vi "Load Settings from XML.vi"(8 "error in (no error)":errorcluster, 11 "Settings in":T1 {"Processing Settings"."Test Parameters"."Allowed Tolerance (%) FS" format="%#_4g"; "Acq Settings"."Config Settings"."Simulated Sensor Injection" scale=0.0..100.0}) -> (0 "error out":errorcluster, 3 "Settings out":T1 {"Processing Settings"."Test Parameters"."Allowed Tolerance (%) FS" format="%#_4g"; "Acq Settings"."Config Settings"."Simulated Sensor Injection" scale=0.0..100.0})   [LabVIEW 2026, in "Settings.lvlib"]
doc: "Attempts to load previous user specified settings from an XML file.\n\nThis VI will not generate an error. If a suitable XML file can't be loaded and parsed then it will simply return the default settings."
uses:
  Settings.lvlib
  <vilib>/Utility/xml.llb/Read From XML File(string).vi
  <vilib>/Utility/xml.llb/Write to XML File(string).vi
  Acquisition/Instrument Specifications Configuration.ctl
  Acquisition/Acquisition.lvlib
  controls/UI/Settings Cluster.ctl
  controls/UI/Measurement Role.ctl
  Acquisition/Instrument Specifications Cluster Configuration.ctl
  controls/UI/Config Settings.ctl
  controls/UI/Acq Settings.ctl
  controls/UI/Units Enum.ctl
  controls/UI/Signal Enum.ctl
  controls/Messaging Payloads/Sensor CoreData Cluster.ctl
  controls/Messaging Payloads/Sensor CoreData.ctl
  Processing/Test Parameters Cluster.ctl
  Processing/Test Parameters.ctl
  Processing/Processing_Engine.lvlib
  controls/UI/Direction.ctl
  controls/UI/Test Sequence Context Cluster.ctl
  controls/UI/Test Sequence Context.ctl
  Processing/Processing Settings.ctl
  controls/UI/Session Identfiers.ctl
  controls/UI/Test Sequence Enum.ctl
  controls/UI/Test Sequence State.ctl
  controls/UI/Test Sequence Settings.ctl
  controls/Controller/Controller Core Data.ctl
  controls/Controller/Stimulus Role.ctl
  controls/Controller/Stimulus Output Configuration.ctl
  controls/Controller/Stimulus Output.ctl
  controls/Controller/Stimulus Outputs.ctl
  controls/Controller/Stimulus Settings.ctl
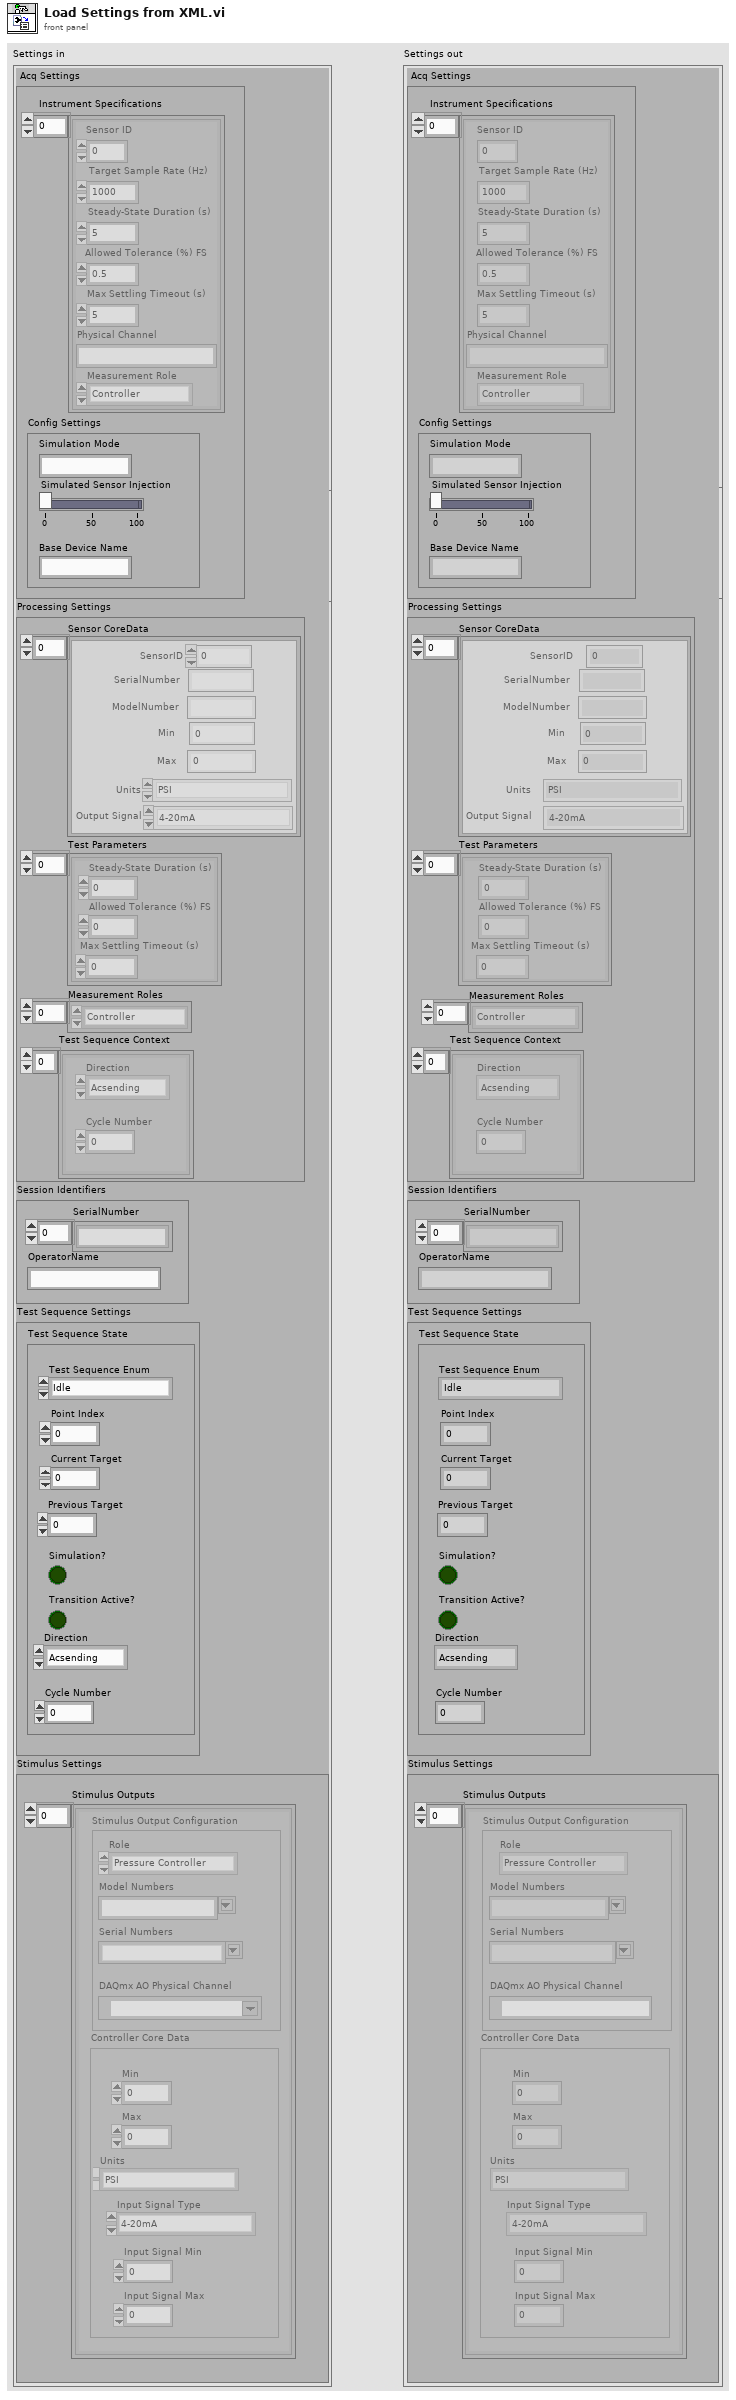
[diagram p1: front panel]
types:
  T1 = typedef "Settings Cluster.ctl" = cluster{"Acq Settings":T2, "Processing Settings":T7, "Session Identifiers":T17, "Test Sequence Settings":T18, "Stimulus Settings":T21}
  T2 = typedef "Acq Settings.ctl" = cluster{"Instrument Specifications":T3, "Config Settings":T6}
  T3 = typedef "Acquisition.lvlib/Instrument Specifications Configuration.ctl" = T4[]
  T4 = typedef "Acquisition.lvlib/Instrument Specifications Cluster Configuration.ctl" = cluster{"Sensor ID":i32, "Target Sample Rate (Hz)":dbl, "Steady-State Duration (s)":i32, "Allowed Tolerance (%) FS":dbl, "Max Settling Timeout (s)":i32, "Physical Channel":string, "Measurement Role":T5}
  T5 = typedef "Settings.lvlib/Measurement Role.ctl" = enum16{"Controller", "Reference", "UUT", "Disable", "All"}
  T6 = typedef "Config Settings.ctl" = cluster{"Simulated Sensor Injection":dbl, "Base Device Name":string, "Simulation Mode":string}
  T7 = typedef "Processing_Engine.lvlib/Processing Settings.ctl" = cluster{"Sensor CoreData":T8, "Test Parameters":T12, "Measurement Roles":T5[], "Test Sequence Context":T14}
  T8 = typedef "Sensor CoreData.ctl" = T9[]
  T9 = typedef "Settings.lvlib/Sensor CoreData Cluster.ctl" = cluster{"SerialNumber":string, "ModelNumber":string, "Min":dbl, "Max":dbl, "Units":T10, "Output Signal":T11, "SensorID":i32}
  T10 = typedef "Units Enum.ctl" = enum16{"PSI", "Deg C", "kPa", "GPM"}
  T11 = typedef "Signal Enum.ctl" = enum16{"4-20mA", "0-10V", "Thermocouple Type K"}
  T12 = typedef "Processing_Engine.lvlib/Test Parameters.ctl" = T13[]
  T13 = typedef "Settings.lvlib/Test Parameters Cluster.ctl" = cluster{"Steady-State Duration (s)":i32, "Allowed Tolerance (%) FS":dbl, "Max Settling Timeout (s)":i32}
  T14 = typedef "Settings.lvlib/Test Sequence Context.ctl" = T15[]
  T15 = typedef "Settings.lvlib/Test Sequence Context Cluster.ctl" = cluster{"Direction":T16, "Cycle Number":i32}
  T16 = typedef "Settings.lvlib/Direction.ctl" = enum16{"Acsending", "Descending"}
  T17 = typedef "Session Identfiers.ctl" = cluster{"SerialNumber":string[], "OperatorName":string}
  T18 = typedef "Test Sequence Settings.ctl" = cluster{"Test Sequence State":T19}
  T19 = typedef "Settings.lvlib/Test Sequence State.ctl" = cluster{"Test Sequence Enum":T20, "Point Index":i32, "Current Target":dbl, "Previous Target":dbl, "Simulation?":bool, "Direction":T16, "Transition Active?":bool, "Cycle Number":i32}
  T20 = typedef "Test Sequence Enum.ctl" = enum16{"Idle", "Start Point", "Point Complete", "Test Complete", "Abort Test", "Reset"}
  T21 = typedef "Settings.lvlib/Stimulus Settings.ctl" = cluster{"Stimulus Outputs":T22}
  T22 = typedef "Settings.lvlib/Stimulus Outputs.ctl" = T23[]
  T23 = typedef "Settings.lvlib/Stimulus Output.ctl" = cluster{"Controller Core Data":T24, "Stimulus Output Configuration":T25}
  T24 = typedef "Settings.lvlib/Controller Core Data.ctl" = cluster{"Min":dbl, "Max":dbl, "Units":T10, "Input Signal Type":T11, "Input Signal Min":dbl, "Input Signal Max":dbl}
  T25 = typedef "Settings.lvlib/Stimulus Output Configuration.ctl" = cluster{"DAQmx AO Physical Channel":tag, "Role":T26, "Model Numbers":string, "Serial Numbers":string}
  T26 = typedef "Stimulus Role.ctl" = enum16{"Pressure Controller", "Temperature Controller"}
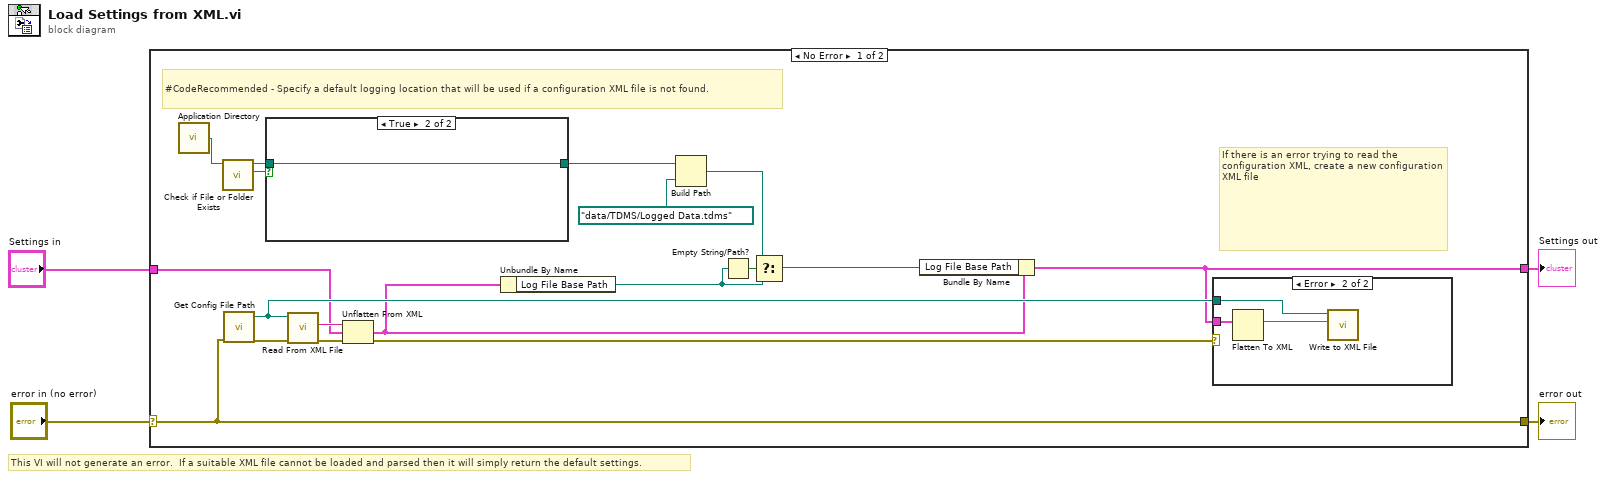
[diagram p0: block diagram]
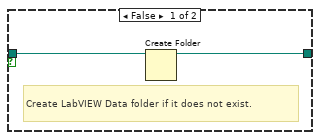
[diagram p2: hidden frame]
diagram:
  # "This VI will not generate an error.  If a suitable XML file cannot be loaded and parsed then it will simply return the default settings."
  n1 = case shown="No Error" "error in (no error)" {
    selector: "error in (no error)" -> [w20 w30]
    tunnel: [w20 w30] -> w3
    tunnel: "Settings in" -> [w15 w29]
    tunnel: [w9 w29] -> w1
    frame No Error {
      # "If there is an error trying to read the configuration XML, create a new configuration XML file"
      # "#CodeRecommended - Specify a default logging location that will be used if a configuration XML file is not found."
      n2 = call <vilib>:"Application Directory.vi"() -> ("Application Directory"=w5:path)
      n3 = call <vilib>:"Check if File or Folder Exists.vi"("path"=w5) -> ("file or folder exists?"=w8:bool, "dup path"=w7:path)  [unwired: 8 in, 1 out]
      n4 = call "Get Config File Path.vi"("error in (no error)"=w20) -> ("error out"=w22:errorcluster, "XML File Path"=w18:path)  [unwired: 9 in]
      n5 = case shown="True" w8 {
        tunnel: w7 -> [w24 w25]
        tunnel: [w23 w25] -> w6
        frame False {
          # "Create LabVIEW Data folder if it does not exist."
          n6 = Create Folder(path (use dialog)=w24) -> (created path=w23:path)  [unwired: 2 in, 2 out]
        }
        frame True {
        }
      }
      n7 = call-poly <vilib>:"Read From XML File.vi"("error in (no error)"=w22, "XML File Path"=w18) -> ("error out"=w17:errorcluster, "XML Elements"=w21:string)  [unwired: 7 in, 1 out]
      n8 = Unflatten From XML(xml string=w21, type=w15, error in (no error)=w17) -> (value=w11:T1, error out=w16:errorcluster)
      n9 = Unbundle By Name(w11) -> ("Log File Base Path"=w13:path)
      n10 = Build Path(base path=w6, name or relative path=path "data/TDMS/Logged Data.tdms" ("App:Default Data Directory")) -> (appended path=w12:path)
      n11 = Empty String/Path?(string/path=w13) -> (empty?=w14:bool)
      n12 = Select(t=w12, s=w14, f=w13) -> (s? t:f=w10:path)
      n13 = Bundle By Name(cluster=w11, "Log File Base Path"=w10) -> (w9:T1)
      n14 = case shown="Error" w16 {
        tunnel: w9 -> [_ w28]
        tunnel: w18 -> [_ w26]
        frame No Error {
        }
        frame Error {
          n15 = Flatten To XML(6:w28) -> (2:w27:string)
          n16 = call-poly <vilib>:"Write to XML File.vi"("XML Input"=w27, "XML File Path"=w26) -> ()  [unwired: 7 in, 3 out]
        }
      }
    }
    frame Error {
    }
  }
  "error out" <- w3
  "Settings out" <- w1
